vi "Instrument Get By ID.vi"(8 "error in (no error)":errorcluster, 10 "sxInstrumentId (\"\")":string, 11 "Connection Refnum":T1) -> (0 "error out":errorcluster, 2 "Instrument Record":T2, 3 "Connection Refnum":T1, 4 "Data Present?":bool)   [LabVIEW 2011]
uses:
  Instrument Record.ctl
  SI.LIB/ODBC/SQL Controls/Connection Refnum.ctl
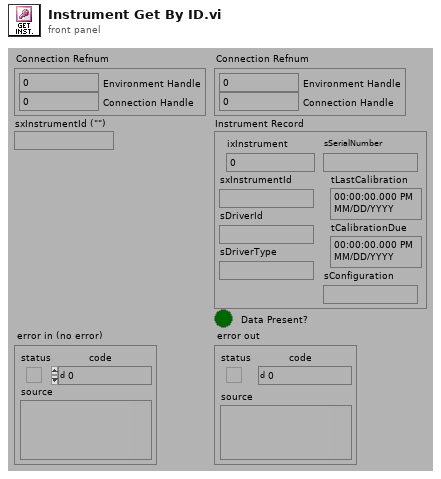
[diagram p1: front panel]
types:
  T1 = typedef "Connection Refnum.ctl" = cluster{"Environment Handle":i32, "Connection Handle":i32}
  T2 = typedef "Instrument Record.ctl" = cluster{"ixInstrument":i32, "sxInstrumentId":string, "sDriverId":string, "sDriverType":string, "sSerialNumber":string, "tLastCalibration":timestamp, "tCalibrationDue":timestamp, "sConfiguration":string}
  T3 = typedef "Statement Refnum.ctl" = cluster{"Statement Handle":i32, "Parameter Number":u16}
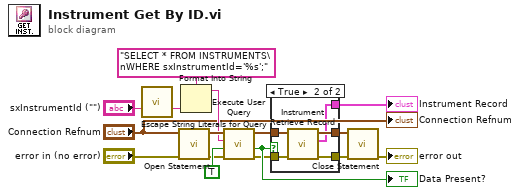
[diagram p0: block diagram]
diagram:
  n1 = call "Escape String Literals for Query.vi"("String"="sxInstrumentId (\"\")") -> ("escaped String"=w2:string)  [unwired: 1 in, 13 out]
  n2 = call "Open Statement.vi"("error in (no error)"="error in (no error)", "Connection Refnum"="Connection Refnum") -> ("error out"=w11:errorcluster, "Statement Refnum"=w12:T3)  [unwired: 4 out]
  n3 = Format Into String(format string="SELECT * FROM INSTRUMENTS\nWHERE sxInstrumentId='%s';" ("Query Name"), w2) -> (resulting string=w8:string)  [unwired: 2 in, 1 out]
  n4 = call "Execute User Query.vi"("error in (no error)"=w11, "Return Data? (f)"=TRUE, "User Query"=w8, "Statement Refnum"=w12) -> ("error out"=w15:errorcluster, "Data Present?"=w16:bool, "Statement Refnum"=w14:T3)  [unwired: 1 out]
  "Data Present?" <- w16
  n5 = case shown="True" w16 {
    tunnel: w15 -> [w17 w23]
    tunnel: w14 -> [w18 w22]
    tunnel: [w17 w20] -> w10
    tunnel: [w18 w21] -> w9
    tunnel: [_ w19] -> w3
    frame False {
    }
    frame True {
      n6 = call "Instrument Retrieve Record.vi"("error in (no error)"=w23, "Statement Refnum"=w22) -> ("error out"=w20:errorcluster, "Instrument"=w19:T2, "Statement Refnum"=w21:T3)  [unwired: 7 out]
    }
  }
  "Instrument Record" <- w3
  n7 = call "Close Statement.vi"("error in (no error)"=w10, "Statement Refnum"=w9) -> ("error out"=→"error out":errorcluster)  [unwired: 5 out]
  "Connection Refnum" <- "Connection Refnum"
